vi "config1.vi"(4 "error in":errorcluster, 5 "ChList":string) -> (0 "error out":errorcluster, 1 "trig":tag, 2 "gps handle":refnum<k15>, 3 "adc handle":refnum<k15>)   [LabVIEW 2010]
uses:
  <instrlib>/niScope/Controls/niScope vertical coupling.ctl
  <instrlib>/niScope/Controls/niScope trigger slope.ctl
  <instrlib>/niScope/Controls/niScope trigger source digital.ctl
  <instrlib>/niScope/Controls/niScope exportable signals.ctl
  <instrlib>/niScope/Controls/niScope export destinations.ctl
  <instrlib>/niSync/niSync.llb/niSync Initialize (IVI).vi
  <instrlib>/niSync/niSync.llb/niSync Set Time Reference (GPS).vi
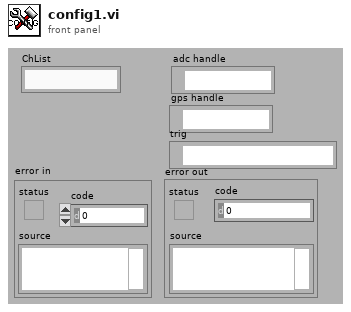
[diagram p1: front panel]
types:
  T1 = typedef "niScope export destinations.ctl" = string
  T2 = typedef "niScope exportable signals.ctl" = u16
  T3 = typedef "niScope trigger source digital.ctl" = string
  T4 = typedef "niScope trigger slope.ctl" = i32
  T5 = typedef "niScope vertical coupling.ctl" = i32
  T6 = cluster{"input impedance":u32, enum16{"1/20", "1/5", "1", "6", "30"}, "vertical coupling":T5, "ChList":string, "min sample rate":dbl, dbl, "min record length":i32, "trigger source":T3, "trigger slope":T4, dbl}
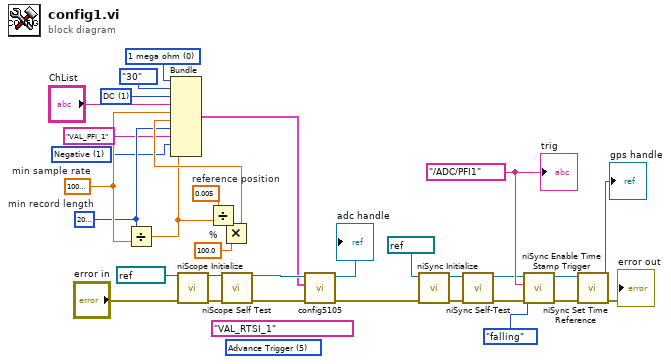
[diagram p0: block diagram]
diagram:
  w27 = 100.0  # %
  w26 = 0.005  # reference position
  (unwired) T1 "VAL_RTSI_1" ("output terminal")
  (unwired) T2 5 items=["None"=0, "Start Trigger"=2, "Advance Trigger"=5, "Reference Trigger"=1, "End of Record Event"=4, "End of Acquisition Event"=3, "Ready for Start Event"=7, "Ready for Advance Event"=6, "Ready for Reference Event"=10, "Reference Clock"=100, "Sample Clock"=101, "5 Volt Power"=13] ("signal")
  w7 = T4 1 items=["Positive", "Negative"] ("trigger slope")
  w30 = tag "/ADC/PFI1" ("terminal")
  w9 = 2000000  # min record length
  w15 = u32 0 items=["1 mega ohm"=0, "50 ohms"=2] ("input impedance")
  w11 = 10000000.0  # min sample rate
  w13 = T5 1 items=["AC", "DC", "Ground"] ("vertical coupling")
  n1 = Divide(x=w9, y=w11) -> (x/y=w6:dbl)
  n2 = call <instrlib>:"niScope Initialize.vi"("resource name"=refnum<k15> "ADC", "error in"="error in") -> ("instrument handle"=w17:refnum<k15>, "error out"=w16:errorcluster)  [unwired: 12 in]
  n3 = Divide(x=w26, y=w6) -> (x/y=w28:dbl)
  n4 = Multiply(x=w28, y=w27) -> (x*y=w10:dbl)
  n5 = Bundle("input impedance"=w15, enum16{"1/20", "1/5", "1", "6", "30"}."30", "vertical coupling"=w13, "ChList"="ChList", "min sample rate"=w11, w10, "min record length"=w9, "trigger source"=T3 "VAL_PFI_1", "trigger slope"=w7, w6) -> (w1:T6)  [unwired: 1 in]
  n6 = call <instrlib>:"niScope Self Test.vi"("instrument handle"=w17, "error in"=w16) -> ("instrument handle out"=w3:refnum<k15>, "error out"=w4:errorcluster)  [unwired: 10 in, 2 out]
  n7 = call "config5105.vi"("error in"=w4, "Cluster"=w1, "instrument handle"=w3) -> ("error out"=w5:errorcluster, "instrument handle out"=→"adc handle":refnum<k15>)  [unwired: 3 in]
  n8 = call-poly <instrlib>:"niSync Initialize.vi"("error in (no error)"=w5, "resource name"=refnum<k15> "GPS") -> ("error out"=w20:errorcluster, "instrument handle out"=w21:refnum<k15>)  [unwired: 8 in]
  n9 = call <instrlib>:"niSync Self-Test.vi"("error in (no error)"=w20, "instrument handle"=w21) -> ("error out"=w18:errorcluster, "instrument handle out"=w19:refnum<k15>)  [unwired: 6 in, 2 out]
  n10 = call <instrlib>:"niSync Enable Time Stamp Trigger.vi"("error in (no error)"=w18, "active edge"=enum32{"rising", "falling", "any"}."falling", "terminal"=w30, "instrument handle"=w19) -> ("error out"=w24:errorcluster, "instrument handle out"=w25:refnum<k15>)  [unwired: 5 in]
  n11 = call-poly <instrlib>:"niSync Set Time Reference.vi"("error in (no error)"=w24, "instrument handle"=w25) -> ("error out"=→"error out":errorcluster, "instrument handle out"=→"gps handle":refnum<k15>)  [unwired: 8 in]
  "trig" <- w30
